vi "HMM.vi"() -> ()   [LabVIEW 2013]
uses:
  <vilib>/Analysis/Matrix/Datatypes/RealMatrix.ctl
  <vilib>/Utility/file.llb/Read From Spreadsheet File (DBL).vi
  <vilib>/Analysis/Matrix/Numeric/Conversions/Matrix To Array - RM.vi
  <vilib>/gmath/NI_Gmath.lvlib
  <vilib>/Analysis/Matrix/NI_Matrix.lvlib
panel:
  out "output":i16[][](array[numeric])
  out "L_k(t)":ext[][](array[numeric])
  out "H_lk":ext[][][](array[numeric])
  out "alk":dbl[][](array[numeric])
  in  "Online_ERP":path=path "C:/Users/Jaehong/Desktop/안전복지프로젝트/LabVIEW/RSVP_offline_onine/분석데이터/140915_전선미/IOHMM/Online_ERP.txt"
  out "covariance matrix_NTERP":T1
  out "STD_NTERP":dbl[](array[numeric])
  out "Average_NTERP":dbl[](array[numeric])
  out "preprocessed_NTERP":dbl[][](array[numeric])
  out "covariance matrix_TERP":T1
  out "STD_TERP":dbl[](array[numeric])
  out "Average_TERP":dbl[](array[numeric])
  out "preprocessed_TERP":dbl[][](array[numeric])
  out "Nontarget_ERP":dbl[][](array[numeric]) format="%0.3f"
  out "Target_ERP":dbl[][](array[numeric]) format="%0.3f"
  in  "Nontarget_Weighted_ERP":path=path "C:/Users/Jaehong/Desktop/안전복지프로젝트/LabVIEW/RSVP_offline_onine/분석데이터/140915_전선미/IOHMM/NonTarget_Weighted_ERP.txt"
  in  "Target_Weighted_ERP":path=path "C:/Users/Jaehong/Desktop/안전복지프로젝트/LabVIEW/RSVP_offline_onine/분석데이터/140915_전선미/IOHMM/Target_Weighted_ERP.txt"
  # "INPUT"
  # "PREPROCESSED"
  # "ITERATION"
  # "OUTPUT"
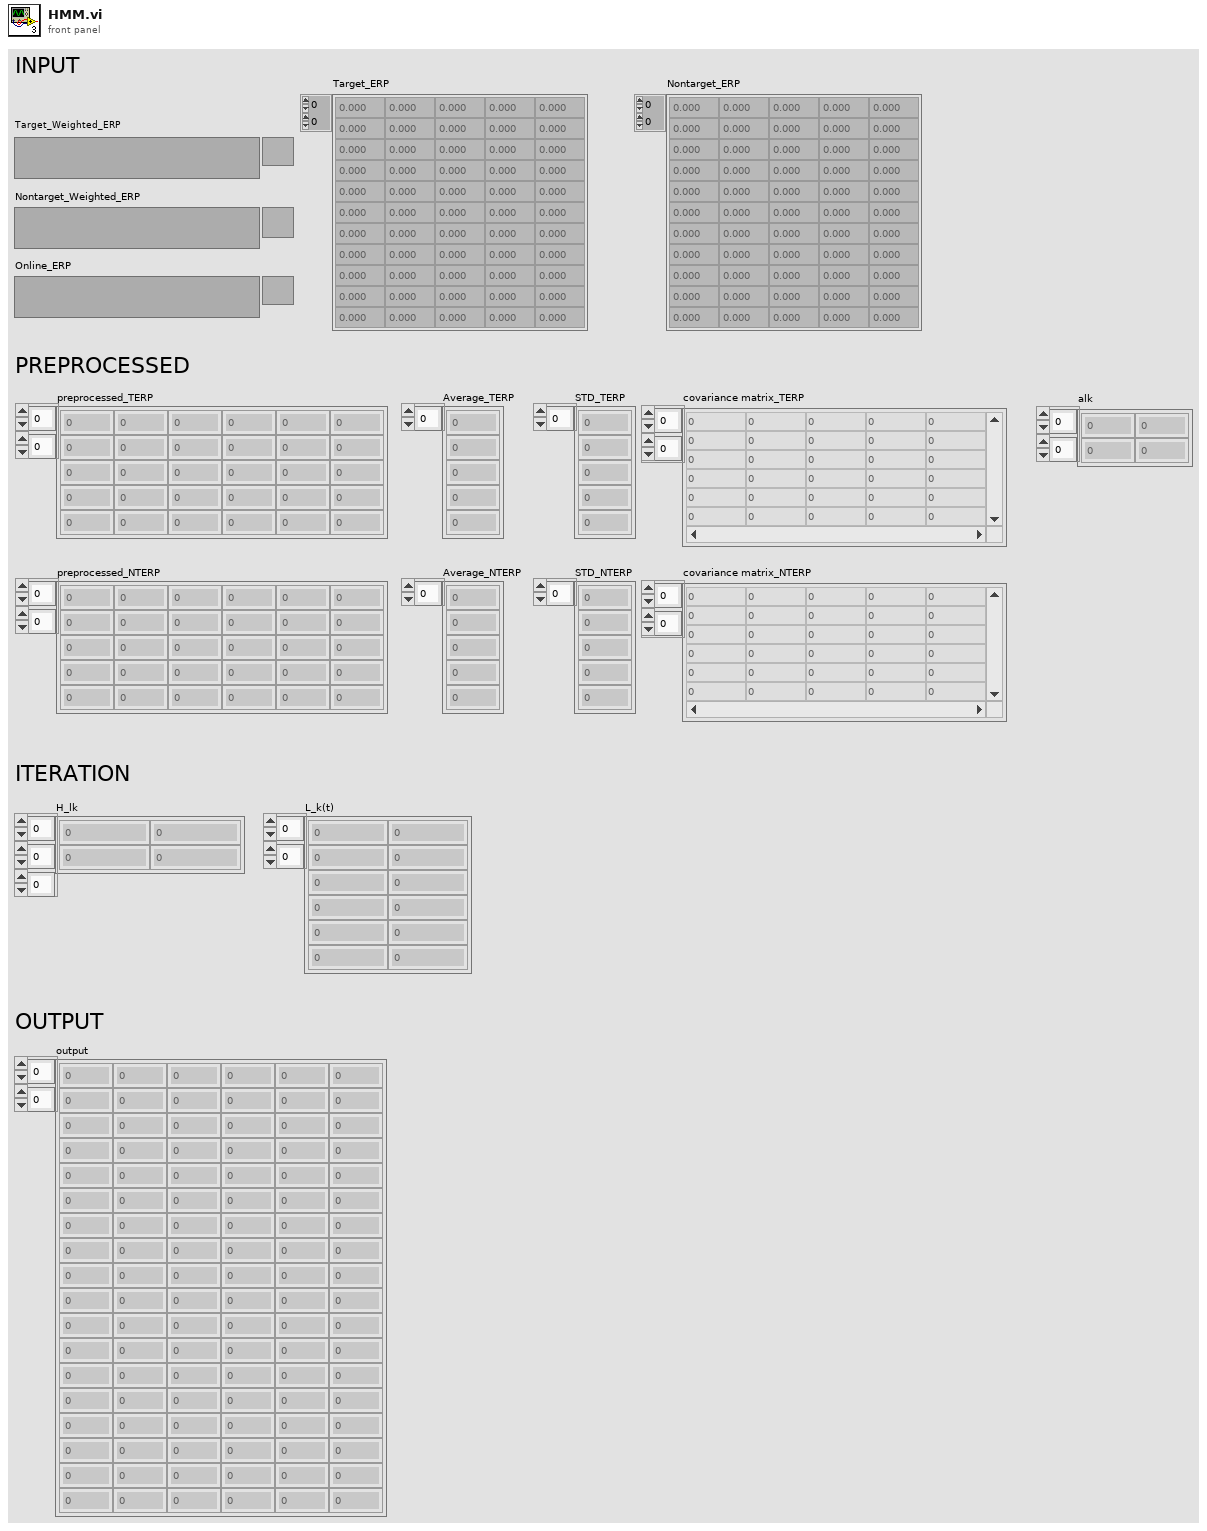
[diagram p1: front panel]
types:
  T1 = typedef "NI_Matrix.lvlib/RealMatrix.ctl" = dbl[][]
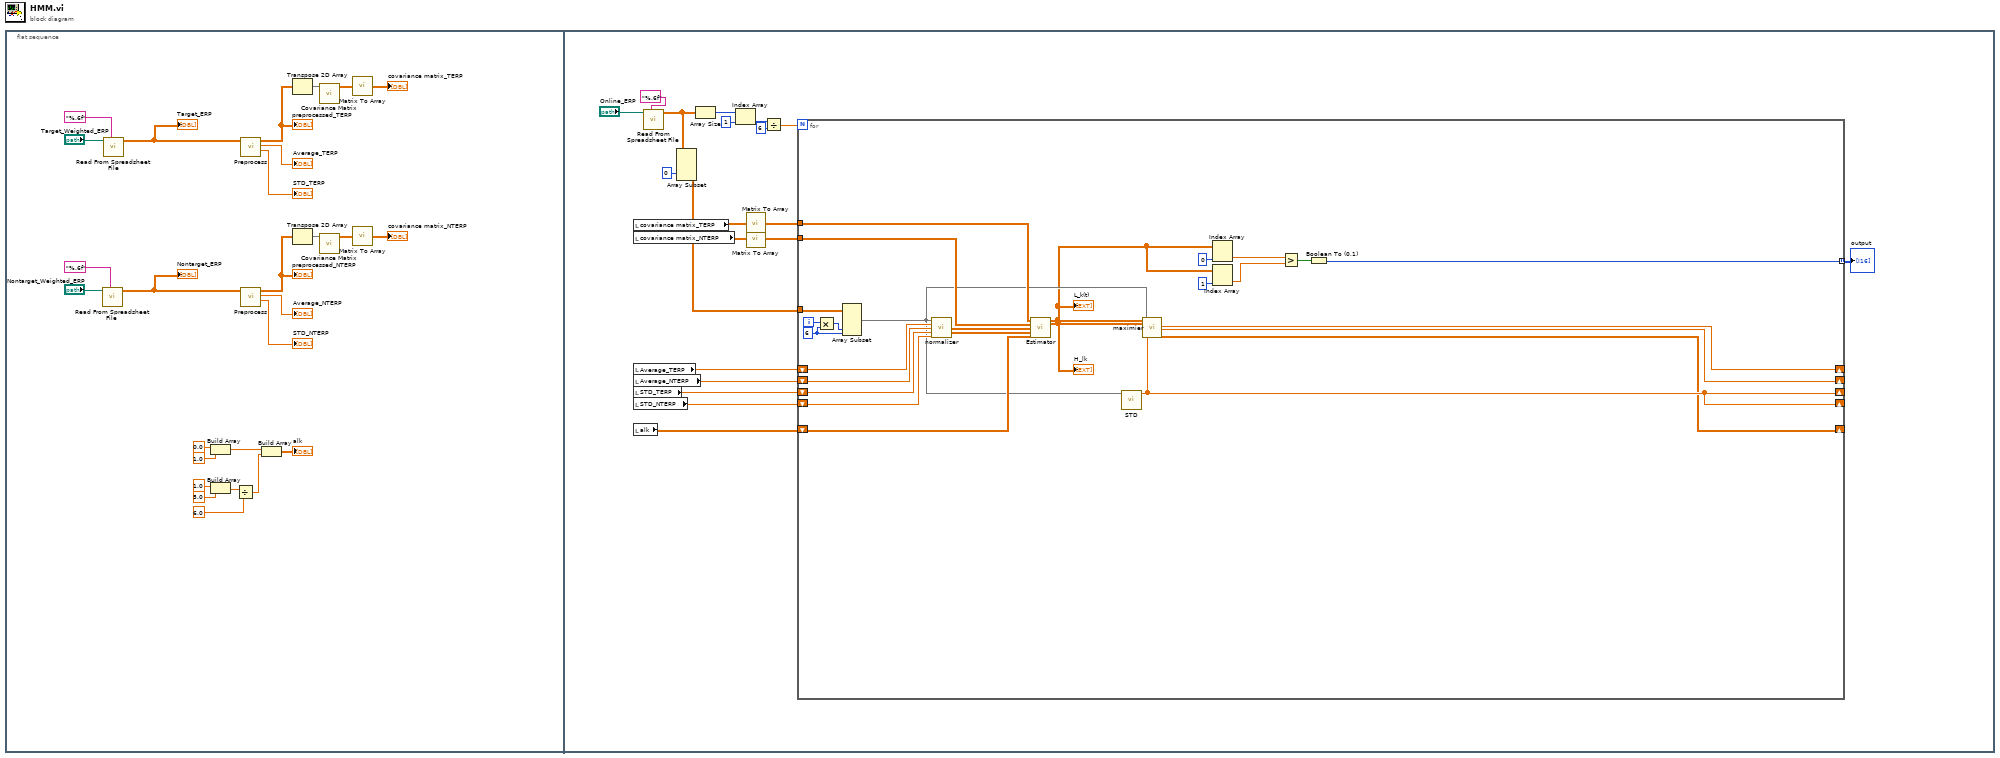
[diagram p0: block diagram]
diagram:
  n1 = flat-sequence {
    frame #0 {
      n2 = call-poly <vilib>:"Read From Spreadsheet File.vi"("format (%.3f)"="%.6f", "file path (dialog if empty)"="Nontarget_Weighted_ERP") -> ("all rows"=w12:dbl[][])  [unwired: 5 in, 4 out]
      "Nontarget_ERP" <- w12
      n3 = call-poly <vilib>:"Read From Spreadsheet File.vi"("format (%.3f)"="%.6f", "file path (dialog if empty)"="Target_Weighted_ERP") -> ("all rows"=w16:dbl[][])  [unwired: 5 in, 4 out]
      "Target_ERP" <- w16
      n4 = Build Array(0.0 ("element"), 1.0 ("element")) -> (w3:dbl[])
      n5 = Build Array(1.0 ("element"), 5.0 ("element")) -> (w4:dbl[])
      n6 = Divide(x=w4, y=6.0) -> (x/y=w2:dbl[])
      n7 = call "Preprocess.vi"("Input(Targter/Nontarget_ERP)"=w16) -> ("STD"=→"STD_TERP":dbl[], "Average"=→"Average_TERP":dbl[], "ouput"=w13:dbl[][])  [unwired: 8 in]
      "preprocessed_TERP" <- w13
      n8 = call "Preprocess.vi"("Input(Targter/Nontarget_ERP)"=w12) -> ("STD"=→"STD_NTERP":dbl[], "Average"=→"Average_NTERP":dbl[], "ouput"=w14:dbl[][])  [unwired: 8 in]
      "preprocessed_NTERP" <- w14
      n9 = Build Array(w3, w2) -> (→"alk":dbl[][])
      n10 = Transpose 2D Array(2D array=w13) -> (transposed array=w22:dbl[][])
      n11 = Transpose 2D Array(2D array=w14) -> (transposed array=w20:dbl[][])
      n12 = call <vilib>:"Covariance Matrix.vi"("X"=w22) -> ("covariance matrix V"=w21:T1)  [unwired: 9 in, 1 out]
      n13 = call <vilib>:"Covariance Matrix.vi"("X"=w20) -> ("covariance matrix V"=w19:T1)  [unwired: 9 in, 1 out]
      n14 = call-poly <vilib>:"Matrix To Array.vi"("Real Matrix"=w21) -> ("Real 2D Array"=→"covariance matrix_TERP":dbl[][])
      n15 = call-poly <vilib>:"Matrix To Array.vi"("Real Matrix"=w19) -> ("Real 2D Array"=→"covariance matrix_NTERP":dbl[][])
    }
    frame #1 {
      n16 = local read "covariance matrix_TERP"() -> (w35:T1)
      n17 = local read "covariance matrix_NTERP"() -> (w34:T1)
      n18 = local read "Average_TERP"() -> (w40:dbl[])
      n19 = local read "Average_NTERP"() -> (w39:dbl[])
      n20 = local read "STD_TERP"() -> (w38:dbl[])
      n21 = local read "STD_NTERP"() -> (w37:dbl[])
      n22 = local read "alk"() -> (w36:dbl[][])
      n23 = call-poly <vilib>:"Read From Spreadsheet File.vi"("format (%.3f)"="%.6f", "file path (dialog if empty)"="Online_ERP") -> ("all rows"=w41:dbl[][])  [unwired: 5 in, 4 out]
      n24 = Array Subset(array=w41, index (col)=0 ("index")) -> (w29:dbl[][])  [unwired: 3 in]
      n25 = Array Size(array=w41) -> (size(s)=w46:i32[])
      n26 = Index Array(array=w46, index=1) -> (element=w44:i32)
      n27 = call-poly <vilib>:"Matrix To Array.vi"("Real Matrix"=w35) -> ("Real 2D Array"=w33:dbl[][])
      n28 = call-poly <vilib>:"Matrix To Array.vi"("Real Matrix"=w34) -> ("Real 2D Array"=w32:dbl[][])
      n29 = Divide(x=w44, y=6) -> (x/y=w42:dbl)
      n30 = for {
        N: w42 -> [_]
        tunnel: w29 -> [w73]
        shift-right: [w58] -> _
        shift-left: w38 -> [w67]
        shift-right: [w58] -> _
        shift-left: w37 -> [w66]
        shift-right: [w57] -> _
        shift-left: w40 -> [w69]
        shift-right: [w56] -> _
        shift-left: w39 -> [w68]
        shift-right: [w55] -> _
        shift-left: w36 -> [w63]
        tunnel: [w48] -> w30 mode=indexing
        tunnel: w33 -> [w62]
        tunnel: w32 -> [w61]
        i -> [w72]
        w71 = 6 ("length")
        n31 = Multiply(x=w72, y=w71) -> (x*y=w70:i32)
        n32 = Array Subset(array=w73, index (col)=w70, length (col)=w71) -> (w59:dbl[][])  [unwired: 2 in]
        n33 = call "normalizer.vi"("online_ERP_raw"=w59, "Average_TERP"=w69, "Average_NTERP"=w68, "STD_TERP"=w67, "STD_NTERP"=w66) -> ("ut_target"=w65:dbl[][], "ut_nontarget"=w64:dbl[][])  [unwired: 9 in]
        n34 = call "Estimator.vi"("target_covariance"=w62, "nontarget_covariance"=w61, "u(t=1, 2, ...6)_target"=w65, "u(t=1, 2, ...6)_nontarget"=w64, "alk"=w63) -> ("L_k(t)"=w54:ext[][], "H_lk"=w60:ext[][][])  [unwired: 9 in]
        "H_lk" <- w60
        "L_k(t)" <- w54
        n35 = call "STD.vi"("Input_array"=w59) -> ("STD"=w58:dbl[])  [unwired: 10 in]
        n36 = call "maximier.vi"("L_k(t)"=w54, "H_lk"=w60, "online_ERP_raw"=w59, "STD"=w58) -> ("Average_TERP"=w57:dbl[], "Average_NTERP"=w56:dbl[], "akl"=w55:ext[][])  [unwired: 11 in, 2 out]
        n37 = Index Array(array=w54, index (col)=0 ("disabled index (col)")) -> (element=w51:ext[])  [unwired: 1 in]
        n38 = Index Array(array=w54, index (col)=1 ("disabled index (col)")) -> (element=w50:ext[])  [unwired: 1 in]
        n39 = Greater?(x=w51, y=w50) -> (0:w49:bool[])
        n40 = Boolean To (0,1)(Boolean=w49) -> (0, 1=w48:i16[])
      }
      "output" <- w30
    }
  }
